vi "Find Origin.vi"(8 "Error In":errorcluster, 11 "Address / Port":i16=1 min=1 max=31 step=1) -> (0 "Error Out":errorcluster, 3 "Address / Port out":i16=1 min=1 max=31 step=1)   [LabVIEW 2014]
doc: "Find the origin of all the motors connected to the ESP300 controller. The base method used to find origin is 1 - Find+0 Position count"
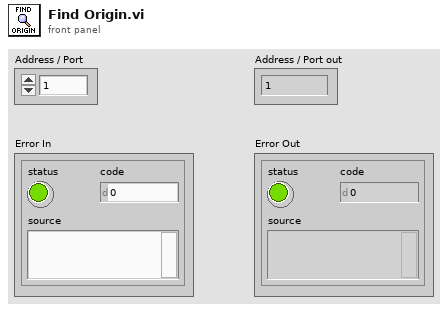
[diagram p1: front panel]
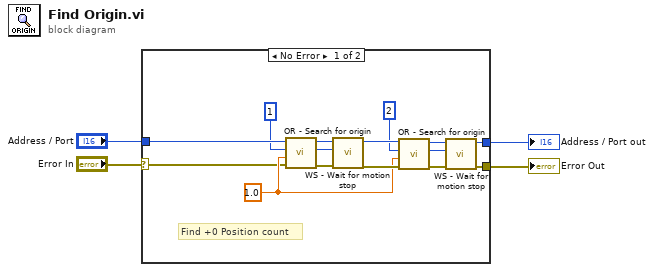
[diagram p0: block diagram]
diagram:
  n1 = case shown="No Error" "Error In" {
    selector: "Error In" -> [w5 w20]
    tunnel: "Address / Port" -> [w16 w21]
    tunnel: [w7 w21] -> w3
    tunnel: [w6 w20] -> w2
    frame No Error {
      w11 = 1.0 ("Type of search")
      # "Find +0 Position count"
      n2 = call "OR - Search for origin.vi"("error in"=w5, "Type of search"=w11, "Axis  #"=i8 1, "Address / Port"=w16) -> ("error out"=w17:errorcluster, "Axis  # out"=w18:i8, "Address / Port out"=w19:i16)  [unwired: 5 in]
      n3 = call "WS - Wait for motion stop.vi"("error in"=w17, "Axis  #"=w18, "Address / Port"=w19) -> ("error out"=w13:errorcluster, "Address / Port dup"=w14:i16)  [unwired: 4 in, 1 out]
      n4 = call "OR - Search for origin.vi"("error in"=w13, "Type of search"=w11, "Axis  #"=i8 2, "Address / Port"=w14) -> ("error out"=w8:errorcluster, "Axis  # out"=w9:i8, "Address / Port out"=w10:i16)  [unwired: 5 in]
      n5 = call "WS - Wait for motion stop.vi"("error in"=w8, "Axis  #"=w9, "Address / Port"=w10) -> ("error out"=w6:errorcluster, "Address / Port dup"=w7:i16)  [unwired: 4 in, 1 out]
    }
    frame Error {
    }
  }
  "Error Out" <- w2
  "Address / Port out" <- w3
